vi "Anritsu VNA Set Trigger Mode.vi"(6 "Channel":i8=1 min=1 max=99 step=1, 7 "Anritsu VNA":T1, 8 "error in (no error)":errorcluster, 10 "Trigger Mode":T2, 11 "VISA Resource Name":refnum<visa-resource-name>) -> (0 "error out":errorcluster, 3 "dup VISA Resource Name":refnum<visa-resource-name>)   [LabVIEW 2011]
doc: "This VI for the HP8753B Network Analyzers reads the stimulus values. Except when performing log sweeps and freq list sweeps, this VI uses the start and stop values and the number of points to calcuate the stimulus values."
uses:
  TypeDefs/Anritsu VNA Trigger Mode.ctl
  TypeDefs/Anritsu VNA Instrument Info.ctl
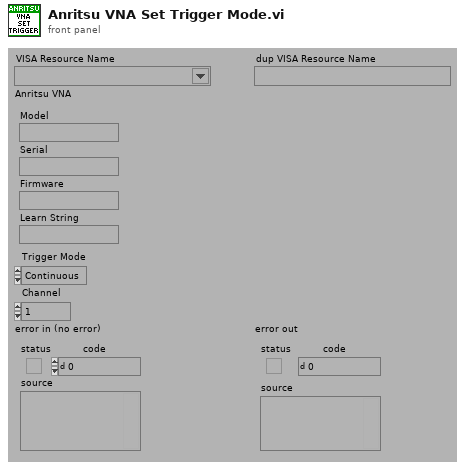
[diagram p1: front panel]
types:
  T1 = typedef "Anritsu VNA Instrument Info.ctl" = cluster{"Model":string, "Serial":string, "Firmware":string, "Learn String":string}
  T2 = typedef "Anritsu VNA Trigger Mode.ctl" = enum16{"Continuous", "Hold", "Single"}
  T3 = typedef "Anritsu VNA Model.ctl" = enum16{"Not Supported", "37XXXX", "MS20XXX", "MS462XX", "MS464XX"}
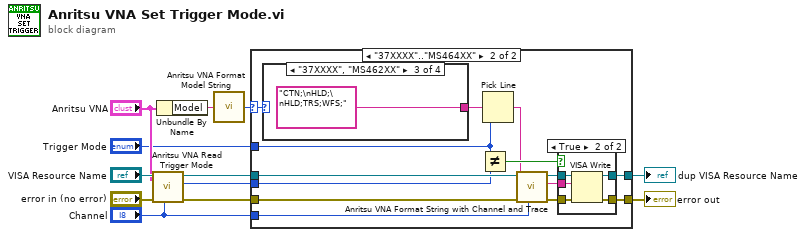
[diagram p0: block diagram]
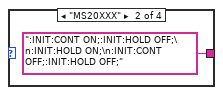
[diagram p4: hidden frame]
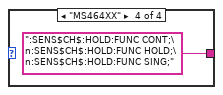
[diagram p5: hidden frame]
diagram:
  n1 = call "Anritsu VNA Read Trigger Mode.vi"("Channel"="Channel", "Anritsu VNA"="Anritsu VNA", "error in (no error)"="error in (no error)", "VISA Resource Name"="VISA Resource Name") -> ("error out"=w7:errorcluster, "Trigger Mode"=w4:T2, "dup VISA Resource Name"=w8:refnum<visa-resource-name>)  [unwired: 5 out]
  n2 = Unbundle By Name("Anritsu VNA") -> ("Model"=w3:string)
  n3 = call "Anritsu VNA Format Model String.vi"("Model"=w3) -> ("Model"=w2:T3)
  n4 = case shown="\"37XXXX\"..\"MS464XX\"" w2 {
    selector: w2 -> [_ w18]
    tunnel: [w14 w26] -> w12
    tunnel: [w13 w25] -> w11
    tunnel: w8 -> [w14 w23]
    tunnel: w7 -> [w13 w22]
    tunnel: "Trigger Mode" -> [_ w20]
    tunnel: w4 -> [_ w19]
    tunnel: "Channel" -> [_ w15]
    frame "Not Supported" {
    }
    frame "37XXXX".."MS464XX" {
      n5 = case shown="\"37XXXX\", \"MS462XX\"" w18 {
        tunnel: [_ ":INIT:CONT ON;:INIT:HOLD OFF;\n:INIT:HOLD ON;\n:INIT:CONT OFF;:INIT:HOLD OFF;" "CTN;\nHLD;\nHLD;TRS;WFS;" ":SENS$CH$:HOLD:FUNC CONT;\n:SENS$CH$:HOLD:FUNC HOLD;\n:SENS$CH$:HOLD:FUNC SING;"] -> w24
        frame "Not Supported" {
        }
        frame "MS20XXX" {
        }
        frame "37XXXX", "MS462XX" {
        }
        frame "MS464XX" {
        }
      }
      n6 = Not Equal?(x=w20, y=w19) -> (x != y?=w21:bool)
      n7 = Pick Line(multi-line string=w24, line index=w20) -> (output string=w16:string)  [unwired: 1 out]
      n8 = call "Anritsu VNA Format String with Channel and Trace.vi"("Channel"=w15, "String"=w16) -> ("String Out"=w17:string)  [unwired: 1 in, 6 out]
      n9 = case shown="True" w21 {
        tunnel: w17 -> [_ w36]
        tunnel: [w31 w35] -> w26
        tunnel: [w30 w34] -> w25
        tunnel: w22 -> [w30 w33]
        tunnel: w23 -> [w31 w32]
        frame False {
        }
        frame True {
          n10 = VISA Write(VISA resource name=w32, write buffer=w36, error in (no error)=w33) -> (VISA resource name out=w35:refnum<visa-resource-name>, error out=w34:errorcluster)  [unwired: 1 out]
        }
      }
    }
  }
  "dup VISA Resource Name" <- w12
  "error out" <- w11
